vi "湿度标定.vi"(0 "温度系数":dbl, 1 "温度波长选择":u8=6 min=1 max=100, 2 "湿度波长选择":u8=9 min=1 max=100, 3 "湿度测量":bool, 5 "初始温度":dbl, 6 "起始湿度":dbl=60.0, 7 "输入数组":dbl[][](array[numeric]), 8 "波长数据":dbl[](array[numeric]), 9 "温度输入":dbl[](array[numeric]), 10 "湿度输入":dbl[](array[numeric]), 17 "湿温比":dbl, 19 "湿度系数":dbl) -> (4 "温度":dbl format="%#_3g", 11 "湿度":dbl format="%#_3g", 12 "湿度":dbl[](graph), 13 "温度":dbl[](graph), 14 "湿度初始波长":dbl format="%#_7g", 15 "湿度变化波长":dbl format="%#.3g", 16 "温度初始波长":dbl format="%#_7g", 18 "输出":dbl[][](array[numeric]))   [LabVIEW 2018]
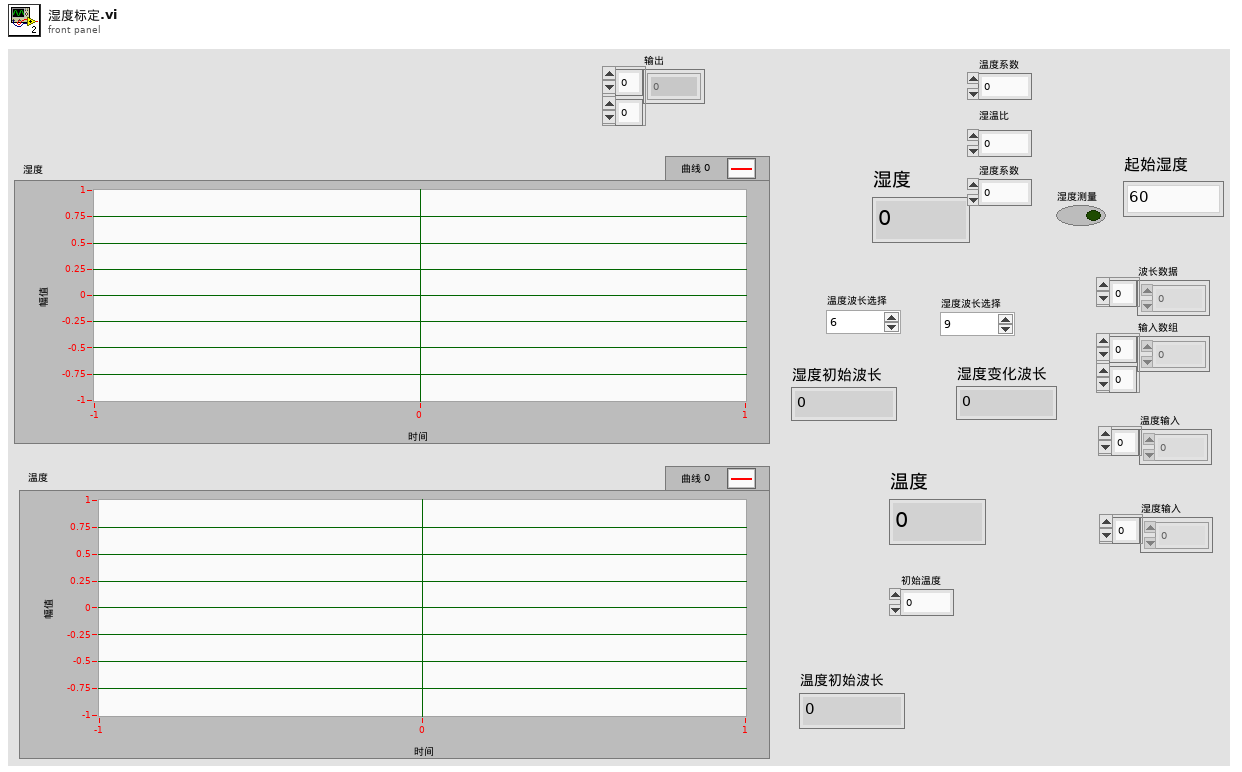
[diagram p1: front panel]
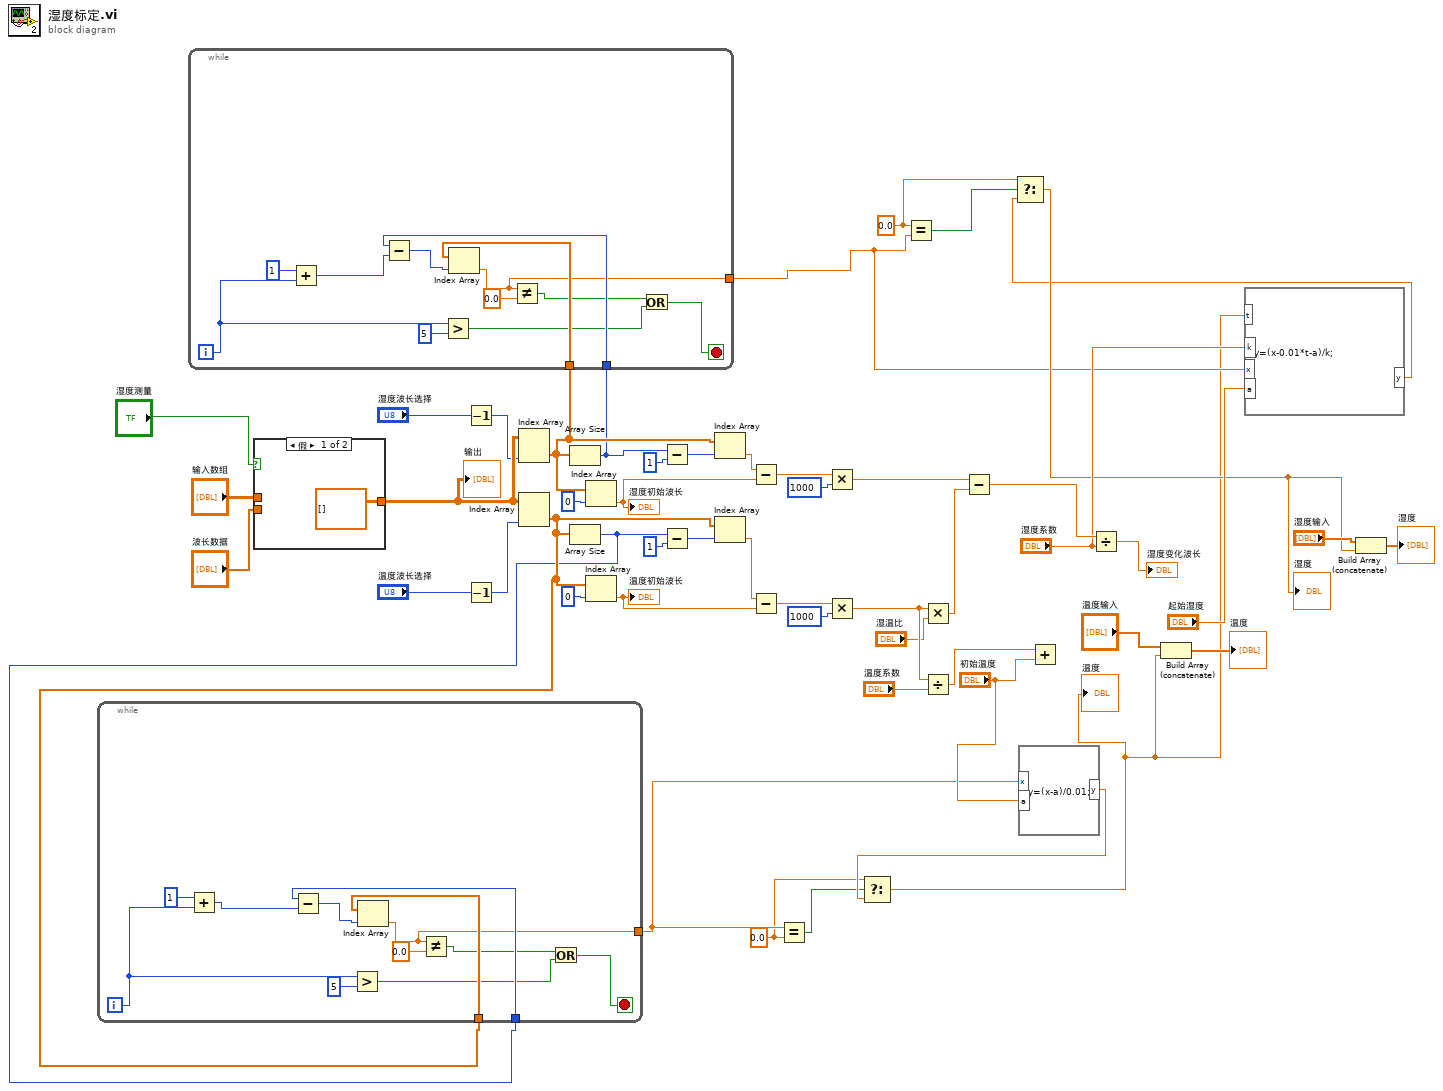
[diagram p0: block diagram]
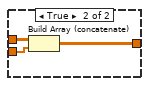
[diagram p2: hidden frame]
diagram:
  w2 = 0.0 ("y")
  w9 = 0.0 ("x")
  n1 = case shown="假" "湿度测量" {
    tunnel: [dbl[][] [] w55] -> w42
    tunnel: "输入数组" -> [_ w54]
    tunnel: "波长数据" -> [_ w53]
    frame False {
    }
    frame True {
      n2 = Build Array (concatenate)(w54, w53) -> (w55:dbl[][])
    }
  }
  "输出" <- w42
  n3 = Decrement(x="湿度波长选择") -> (x-1=w36:u8)
  n4 = Decrement(x="温度波长选择") -> (x-1=w35:u8)
  n5 = Index Array(array=w42, index (col)=w36) -> (element=w15:dbl[])  [unwired: 1 in]
  n6 = Index Array(array=w42, index (col)=w35) -> (element=w13:dbl[])  [unwired: 1 in]
  n7 = Array Size(array=w15) -> (size(s)=w14:i32)
  n8 = while {
    tunnel: w14 -> [w67]
    tunnel: w15 -> [w65]
    tunnel: [w60] -> w6
    i -> [w59]
    stop <- w56 stop-if-true
    n9 = Add(x=1, y=w59) -> (x+y=w57:i32)
    n10 = Subtract(x=w67, y=w57) -> (x-y=w66:i32)
    n11 = Greater?(x=w59, y=5) -> (0:w61:bool)
    n12 = Index Array(array=w65, index=w66) -> (element=w60:dbl)
    n13 = Not Equal?(x=w60, y=0.0) -> (x != y?=w62:bool)
    n14 = Or(x=w62, y=w61) -> (x .or. y?=w56:bool)
  }
  n15 = Array Size(array=w13) -> (size(s)=w12:i32)
  n16 = while {
    tunnel: w12 -> [w79]
    tunnel: w13 -> [w77]
    tunnel: [w72] -> w4
    i -> [w71]
    stop <- w68 stop-if-true
    n17 = Add(x=1, y=w71) -> (x+y=w69:i32)
    n18 = Subtract(x=w79, y=w69) -> (x-y=w78:i32)
    n19 = Greater?(x=w71, y=5) -> (0:w73:bool)
    n20 = Index Array(array=w77, index=w78) -> (element=w72:dbl)
    n21 = Not Equal?(x=w72, y=0.0) -> (x != y?=w74:bool)
    n22 = Or(x=w74, y=w73) -> (x .or. y?=w68:bool)
  }
  n23 = Index Array(array=w15, index=0 ("y")) -> (element=w41:dbl)
  "湿度初始波长" <- w41
  n24 = Index Array(array=w13, index=0 ("y")) -> (element=w31:dbl)
  "温度初始波长" <- w31
  n25 = Subtract(x=w14, y=1) -> (x-y=w45:i32)
  n26 = Subtract(x=w12, y=1) -> (x-y=w50:i32)
  n27 = Index Array(array=w15, index=w45) -> (element=w16:dbl)
  n28 = Index Array(array=w13, index=w50) -> (element=w17:dbl)
  n29 = Subtract(x=w16, y=w41) -> (x-y=w39:dbl)
  n30 = Subtract(x=w17, y=w31) -> (x-y=w30:dbl)
  n31 = Equal?(x=w4, y=w2) -> (x = y?=w3:bool)
  n32 = Multiply(x=w39, y=1000) -> (x*y=w40:dbl)
  n33 = Multiply(x=w30, y=1000) -> (x*y=w26:dbl)
  n34 = Equal?(x=w9, y=w6) -> (x = y?=w10:bool)
  n35 = Multiply(x=w26, y="湿温比") -> (x*y=w25:dbl)
  n36 = Divide(x=w26, y="温度系数") -> (x/y=w27:dbl)
  n37 = Subtract(x=w40, y=w25) -> (x-y=w22:dbl)
  n38 = formula code="y=(x-a)/0.01;"("x"=w4, "a"="初始温度") -> ("y"=w5:dbl)
  n39 = Select(t=w2, s=w3, f=w5) -> (s? t:f=w1:dbl)
  "温度" <- w1
  n40 = Add(x=w27, y="初始温度") -> ()  [unwired: 1 out]
  n41 = Divide(x=w22, y="湿度系数") -> (x/y=→"湿度变化波长":dbl)
  n42 = Build Array (concatenate)("温度输入", w1) -> (→"温度":dbl[])
  n43 = formula code="y=(x-0.01*t-a)/k;"("x"=w6, "a"="起始湿度", "k"="湿度系数", "t"=w1) -> ("y"=w7:dbl)
  n44 = Select(t=w9, s=w10, f=w7) -> (s? t:f=w8:dbl)
  "湿度" <- w8
  n45 = Build Array (concatenate)("湿度输入", w8) -> (→"湿度":dbl[])
